vi "Data_Add_Frame.vi"(7 "color(black)":u32(colorbox)=51261, 8 "error in (no error)":errorcluster caption="错误输入（无错误）", 9 "pen":T1={"Width"=1, "Style"=enum."Solid"}, 10 "Width":i16, 11 "Picture_Class 输入":refnum<class "Picture_Class.lvclass"> caption="DNL_LabVIEW Object in") -> (0 "error out":errorcluster caption="错误输出", 3 "Picture_Class 输出":refnum<class "Picture_Class.lvclass"> caption="DNL_LabVIEW Object out")   [LabVIEW 2013, in "Picture_Class.lvclass"]
uses:
  Picture_Class.lvclass
  Picture_Class.lvclass/Picture_Class.ctl
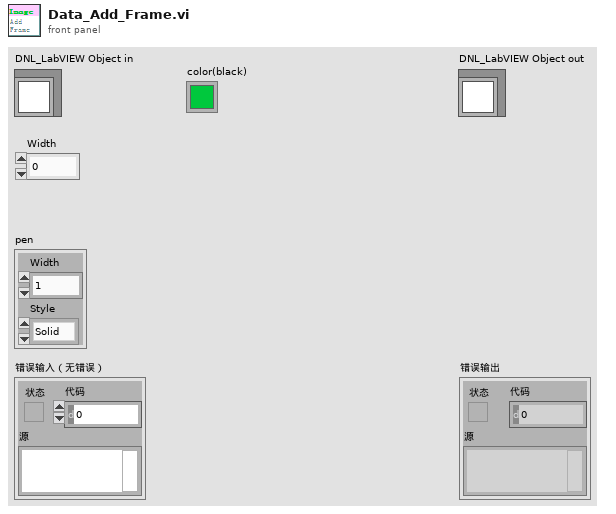
[diagram p1: front panel]
types:
  T1 = cluster{"Width":i16, "Style":enum32{"Solid", "Dash", "Dot", "DashDot", "DashDotDot"}}
  T2 = typedef "imagedata.ctl" = cluster{"image type":i32, "image depth":i32, "image":u8[], "mask":u8[], "colors":u32[], "Rectangle":cluster{"left":i16, "top":i16, "right":i16, "bottom":i16}}
  T3 = cluster{"left":i16, "top":i16, "right":i16, "bottom":i16}
  T4 = typedef "LVBoundsTypeDef.ctl" = cluster{"Width":u32, "Height":u32}
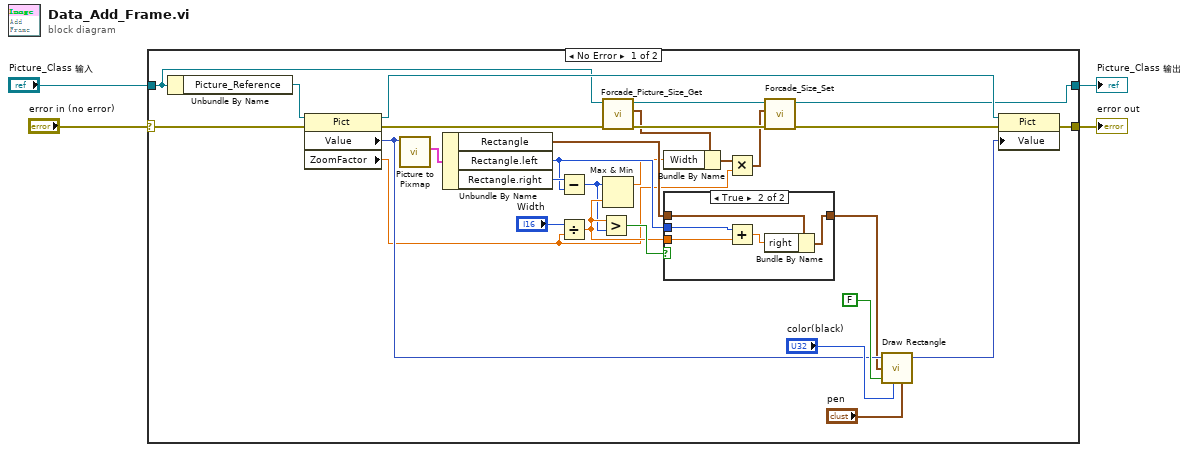
[diagram p0: block diagram]
diagram:
  n1 = case shown="No Error" "error in (no error)" {
    selector: "error in (no error)" -> [w32 w41]
    tunnel: [w22 w41] -> w3
    tunnel: [w17 w40] -> w1
    tunnel: "Picture_Class 输入" -> [w15 w40]
    frame No Error {
      n2 = Unbundle By Name(w15) -> ("Picture_Reference"=w33:refnum<vi>)
      n3 = property class="Pict"(reference=w33, error in=w32) -> (reference out=w23:refnum<vi>, error out=w13:errorcluster, "Value"=w28:picture, "ZoomFactor"=w5:sgl)
      n4 = call <vilib>:"Picture to Pixmap.vi"("picture"=w28) -> ("image data"=w27:T2)  [unwired: 9 in, 1 out]
      n5 = Unbundle By Name(w27) -> ("Rectangle"=w26:T3, "Rectangle.left"=w18:i16, "Rectangle.right"=w19:i16)
      n6 = Subtract(x=w19, y=w18) -> (x-y=w8:i16)
      n7 = Divide(x="Width", y=w5) -> (x/y=w9:sgl)
      n8 = Greater?(x=w9, y=w8) -> (0:w20:bool)
      n9 = call "Forcade_Picture_Size_Get.vi"("error in (no error)"=w13, "Picture_Class 输入"=w15) -> ("error out"=w12:errorcluster, "Picture Size"=w11:T4, "Picture_Class 输出"=w14:refnum<class "Picture_Class.lvclass">)  [unwired: 7 in]
      n10 = Max & Min(x=w8, y=w9) -> (max(x,y)=w7:sgl)  [unwired: 1 out]
      n11 = Bundle By Name(cluster=w11, "Width"=w7) -> (w10:T4)
      n12 = case shown="True" w20 {
        tunnel: w26 -> [w34 w39]
        tunnel: [w34 w38] -> w25
        tunnel: w18 -> [_ w37]
        tunnel: w9 -> [_ w36]
        frame False {
        }
        frame True {
          n13 = Add(x=w37, y=w36) -> (x+y=w35:sgl)
          n14 = Bundle By Name(cluster=w39, "right"=w35) -> (w38:T3)
        }
      }
      n15 = Multiply(x=w10, y=w5) -> (x*y=w6:cluster{"Width":sgl, "Height":sgl})
      n16 = call "Forcade_Size_Set.vi"("error in (no error)"=w12, "Draw Area Size"=w6, "Picture_Class 输入"=w14) -> ("error out"=w16:errorcluster, "Picture_Class 输出"=w17:refnum<class "Picture_Class.lvclass">)  [unwired: 7 in]
      n17 = call <vilib>:"Draw Rectangle.vi"("picture"=w28, "rect"=w25, "fill?(F)"=FALSE, "color(black)"="color(black)", "pen"="pen") -> ("new picture"=w24:picture)  [unwired: 4 in]
      n18 = property class="Pict"(reference=w23, error in=w16, "Value"=w24) -> (error out=w22:errorcluster)  [unwired: 1 out]
    }
    frame Error {
    }
  }
  "error out" <- w3
  "Picture_Class 输出" <- w1
